vi "string keine Sonderzeichen.vi"(7 "String in":string) -> (8 "trimmed string":string caption="Gekürzter String")   [LabVIEW 2017, in "util.lvlib"]
uses:
  util.lvlib
  <vilib>/regexp/Match Regular Expression.xnode
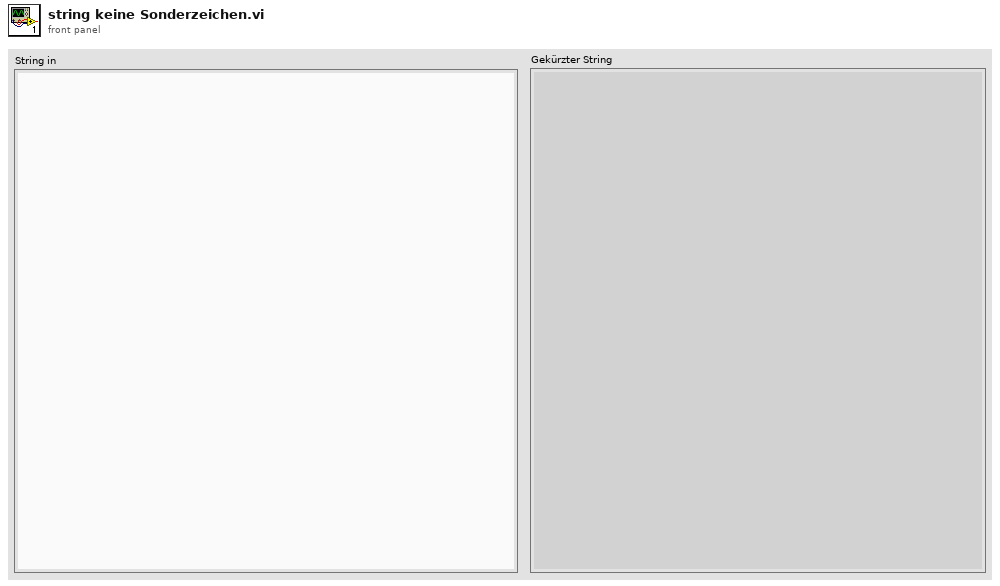
[diagram p1: front panel]
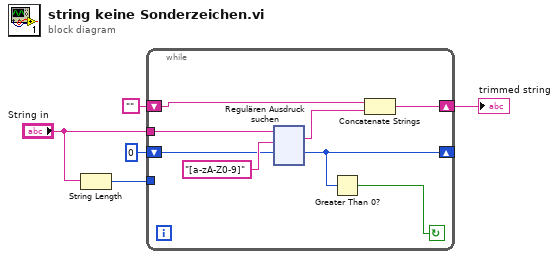
[diagram p0: block diagram]
diagram:
  n1 = String Length(string="String in") -> (length=w4:i32)
  n2 = while {
    tunnel: "String in" -> [w12]
    tunnel: w4 -> [_]
    shift-right: [w7] -> _
    shift-left: 0 ("Offset nach Übereinstimmung") -> [w8]
    shift-right: [w10] -> w1
    shift-left: "" -> [w9]
    stop <- w6 continue-if-true
    n3 = xnode "Regulären Ausdruck suchen"("input string"=w12, "regular expression"="[a-zA-Z0-9]" ("Regulärer Ausdruck"), "offset (0)"=w8) -> ("whole match"=w11:string, "offset past match"=w7:i32)  [unwired: 3 in, 3 out]
    n4 = Greater Than 0?(x=w7) -> (x > 0?=w6:bool)
    n5 = Concatenate Strings(w9, w11) -> (w10:string)
  }
  "trimmed string" <- w1
